vi "ACQuire_COUNt.vi"(7 "Write?":bool, 8 "Error":errorcluster caption="错误输入（无错误）", 10 "Count":u32, 11 "VISA resource name":refnum<visa-resource-name>) -> (0 "Error out":errorcluster, 2 "Count out":u32, 3 "VISA resource name out":refnum<visa-resource-name>)   [LabVIEW 2020]
doc: "每个包的数量"
panel:
  out "读取缓冲区":string
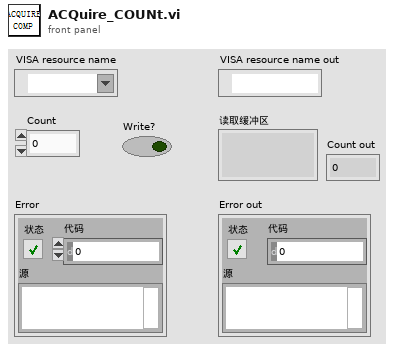
[diagram p1: front panel]
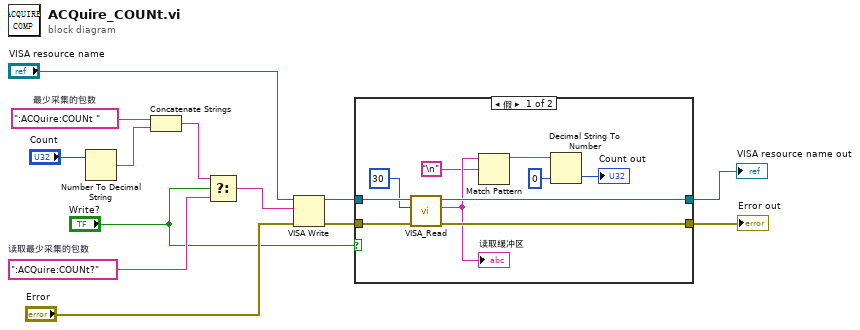
[diagram p0: block diagram]
diagram:
  w10 = ":ACQuire:COUNt?"  # 读取最少采集的包数
  w12 = ":ACQuire:COUNt "  # 最少采集的包数
  n1 = Number To Decimal String(number="Count") -> (decimal integer string=w2:string)  [unwired: 1 in]
  n2 = Concatenate Strings(w12, w2) -> (w11:string)
  n3 = Select(t=w11, s="Write?", f=w10) -> (s? t:f=w9:string)
  n4 = VISA Write(VISA resource name="VISA resource name", write buffer=w9, error in (no error)="Error") -> (VISA resource name out=w5:refnum<visa-resource-name>, error out=w7:errorcluster)  [unwired: 1 out]
  n5 = case shown="假" "Write?" {
    tunnel: w5 -> [w23 w25]
    tunnel: w7 -> [w22 w24]
    tunnel: [w20 w24] -> w6
    tunnel: [w21 w25] -> w3
    frame False {
      n6 = call "VISA_Read.vi"("Error"=w22, "字节总数"=u32 30, "VISA resource name"=w23) -> ("Error out"=w20:errorcluster, "读取缓冲区"=w19:string, "VISA resource name out"=w21:refnum<visa-resource-name>)  [unwired: 6 in]
      "读取缓冲区" <- w19
      n7 = Match Pattern(string=w19, regular expression="\n") -> (before substring=w16:string)  [unwired: 1 in, 3 out]
      n8 = Decimal String To Number(string=w16, default (0L)=u32 0 ("默认(0 I32)")) -> (number=→"Count out":u32)  [unwired: 1 in, 1 out]
    }
    frame True {
    }
  }
  "VISA resource name out" <- w3
  "Error out" <- w6
